vi "Que_Destroy.vi"(8 "error in (no error)":errorcluster caption="error in", 11 "QueeuName":string) -> (0 "error out":errorcluster)   [LabVIEW 2016]
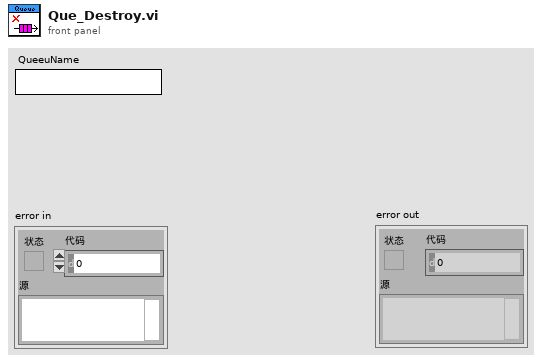
[diagram p1: front panel]
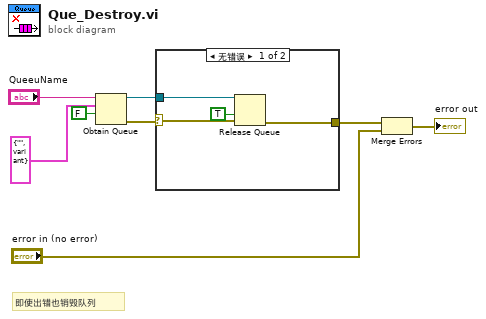
[diagram p0: block diagram]
diagram:
  # "即使出错也销毁队列"
  n1 = Obtain Queue(name (unnamed)="QueeuName", element data type=cluster{string, "变体":variant} {"", "变体"=variant}, create if not found? (T)=FALSE ("如未找到是否创建？(T)")) -> (queue out=w1:refnum<queue>, error out=w7:errorcluster)  [unwired: 2 in, 1 out]
  n2 = case shown="无错误" w7 {
    selector: w7 -> [w12 w13]
    tunnel: w1 -> [w10 _]
    tunnel: [w9 w13] -> w4
    frame No Error {
      n3 = Release Queue(queue=w10, force destroy? (F)=TRUE ("强制销毁？(F)"), error in (no error)=w12) -> (error out=w9:errorcluster)  [unwired: 2 out]
    }
    frame Error {
    }
  }
  n4 = Merge Errors(w4, "error in (no error)") -> (→"error out":errorcluster)
